vi "FTW-File-TextWrite.vi"(0 "Filepath":path, 5 "Text to Write":string, 7 "Mode":enum16{"Overwrite", "Append"}(ring), 11 "error in":errorcluster) -> (4 "Filepath out":path, 15 "error out":errorcluster)   [LabVIEW 2013]
panel:
  # "Inputs"
  # "Outputs"
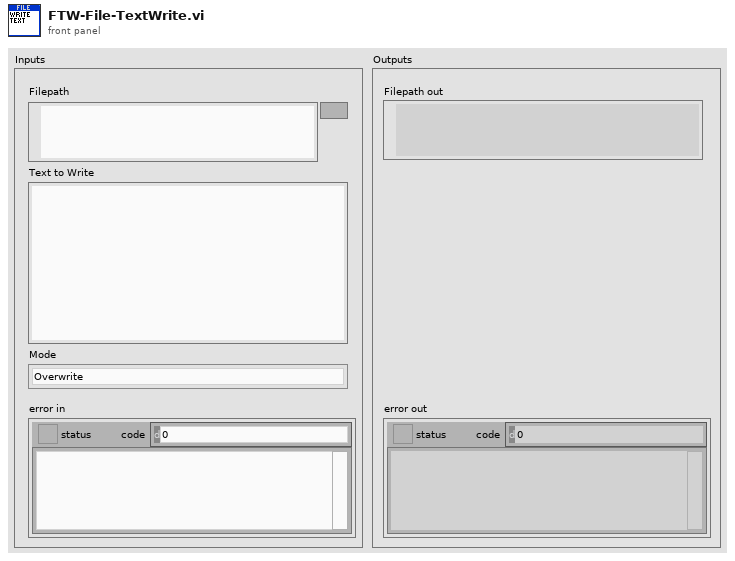
[diagram p1: front panel]
types:
  T1 = enum16{"open", "replace", "create", "open or create", "replace or create", "replace or create with confirmation"}
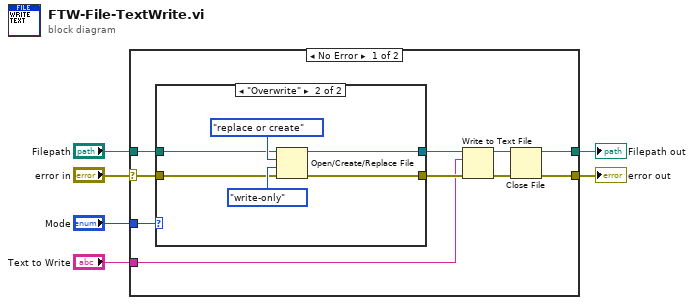
[diagram p0: block diagram]
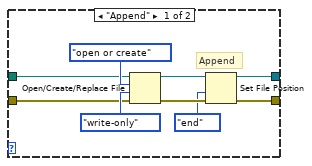
[diagram p2: hidden frame]
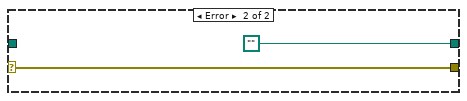
[diagram p3: hidden frame]
diagram:
  n1 = case shown="No Error" "error in" {
    selector: "error in" -> [w7 w32]
    tunnel: "Text to Write" -> [w12 _]
    tunnel: "Filepath" -> [w11 _]
    tunnel: [w10 path ""] -> w4
    tunnel: [w9 w32] -> w3
    tunnel: "Mode" -> [w8 _]
    frame No Error {
      n2 = case shown="\"Overwrite\"" w8 {
        tunnel: [w21 w26] -> w14
        tunnel: [w20 w27] -> w13
        tunnel: w11 -> [w18 w29]
        tunnel: w7 -> [w17 w28]
        frame "Append" {
          # "Append"
          n3 = Open/Create/Replace File(file path (use dialog)=w18, error in=w17, operation (0:open)=T1."open or create", access (0:read/write)=enum16{"read/write", "read-only", "write-only"}."write-only") -> (refnum out=w23:refnum<file>, error out=w22:errorcluster)  [unwired: 2 in, 1 out]
          n4 = Set File Position(refnum=w23, from (0:start)=enum16{"start", "end", "current"}."end", error in=w22) -> (refnum out=w20:refnum<file>, error out=w21:errorcluster)  [unwired: 1 in]
        }
        frame "Overwrite" {
          n5 = Open/Create/Replace File(file path (use dialog)=w29, error in=w28, operation (0:open)=T1."replace or create", access (0:read/write)=enum16{"read/write", "read-only", "write-only"}."write-only") -> (refnum out=w27:refnum<file>, error out=w26:errorcluster)  [unwired: 2 in, 1 out]
        }
      }
      n6 = Write to Text File(file (use dialog)=w13, text=w12, error in=w14) -> (refnum out=w16:refnum<file>, error out=w15:errorcluster)  [unwired: 1 in, 1 out]
      n7 = Close File(refnum=w16, error in=w15) -> (path=w10:path, error out=w9:errorcluster)
    }
    frame Error {
    }
  }
  "error out" <- w3
  "Filepath out" <- w4
